vi "BRig_dataRT_stats__nReward_right.vi"() -> (2 "output_nReward_right":i32)   [LabVIEW 2014]
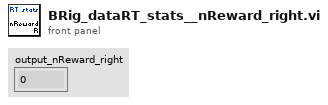
[diagram p1: front panel]
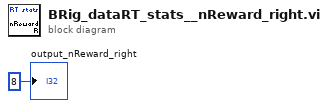
[diagram p0: block diagram]
diagram:
  "output_nReward_right" <- 8 ("output_iBlock")
